vi "light_clock_data.vi"(11 "Pixel Colors":u32[](array[colorbox])) -> ()   [LabVIEW 2011]
uses:
  <vilib>/Rock Robotics/WPI/SPI/WPI_SPIDevRef.ctl
  <vilib>/vision/NI_Vision_Development_Module.lvlib
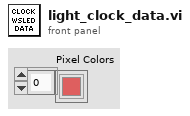
[diagram p1: front panel]
types:
  T1 = typedef "WPI_SPIDevRef.ctl" = cluster{"DevStatus":errorcluster}
  T2 = cluster{"Red (or Hue) value":u8, "Green (or Sat) value":u8, "Blue (or Light or Val) value":u8}
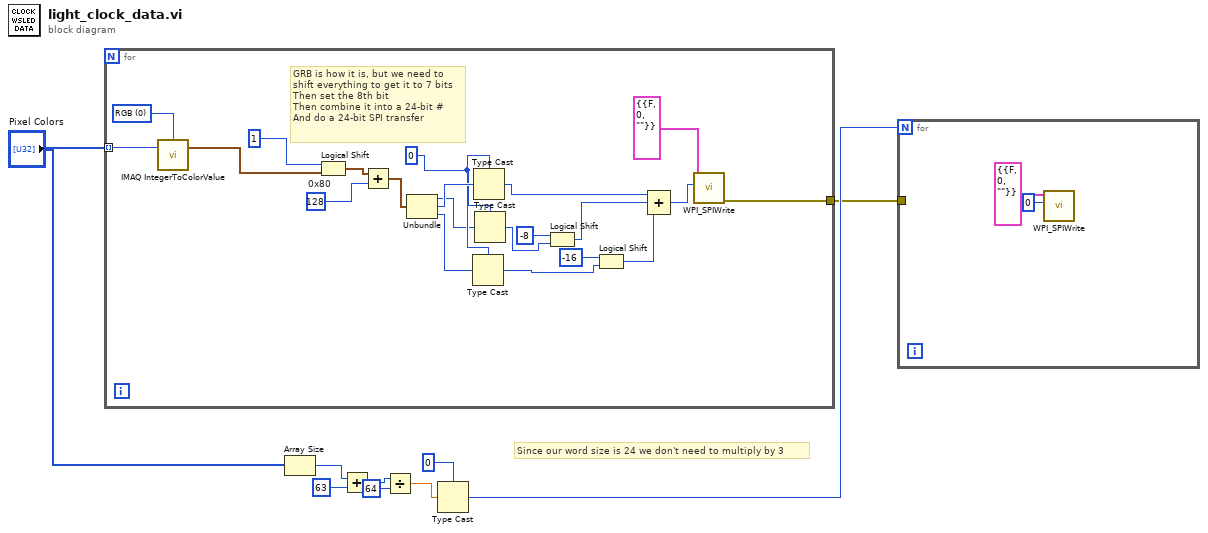
[diagram p0: block diagram]
diagram:
  # "Since our word size is 24 we don't need to multiply by 3"
  n1 = for {
    tunnel: "Pixel Colors" -> [w30] mode=indexing
    tunnel: [w10] -> w1
    w16 = u32 0
    w25 = u8 128  # 0x80
    w29 = u16 0 items=["RGB", "HSL", "HSV", "HSI"] ("Color Mode")
    # "GRB is how it is, but we need to\nshift everything to get it to 7 bits\nThen set the 8th bit\nThen combine it into a 24-bit #\nAnd do a 24-bit SPI transfer"
    n2 = call "IMAQ IntegerToColorValue"("U32 value"=w30, "Color Mode"=w29) -> ("Color Value"=w27:T2)  [unwired: 3 in, 3 out]
    n3 = Logical Shift(y=1, x=w27) -> (x << y=w26:T2)
    n4 = Add(x=w26, y=w25) -> (x+y=w19:T2)
    n5 = Unbundle(w19) -> ("Red (or Hue) value"=w15:u8, "Green (or Sat) value"=w18:u8, "Blue (or Light or Val) value"=w14:u8)
    n6 = Type Cast(type=w16, x=w14) -> (*(type *) &x=w12:u32)
    n7 = Type Cast(type=w16, x=w18) -> (*(type *) &x=w17:u32)
    n8 = Type Cast(type=w16, x=w15) -> (*(type *) &x=w13:u32)
    n9 = Logical Shift(y=i8 -8, x=w13) -> (x << y=w23:u32)
    n10 = Logical Shift(y=i8 -16, x=w12) -> (x << y=w22:u32)
    n11 = Compound Arithmetic op=ADD(w17, w23, w22) -> (w20:u32)
    n12 = call <vilib>:"WPI_SPIWrite.vi"("Data To Send"=w20, "SPIDevRef"=T1 {"DevStatus"={"status"=FALSE, "code"=0, "source"=""}}) -> ("error out"=w10:errorcluster)  [unwired: 8 in, 1 out]
  }
  n13 = Array Size(array="Pixel Colors") -> (size(s)=w8:i32)
  n14 = Add(x=w8, y=63) -> (x+y=w6:i32)
  n15 = Divide(x=w6, y=64) -> (x/y=w4:dbl)
  n16 = Type Cast(type=0 ("y"), x=w4) -> (*(type *) &x=w2:i32)
  n17 = for {
    N: w2 -> [_]
    tunnel: w1 -> [_]
    n18 = call <vilib>:"WPI_SPIWrite.vi"("Data To Send"=u32 0, "SPIDevRef"=T1 {"DevStatus"={"status"=FALSE, "code"=0, "source"=""}}) -> ()  [unwired: 8 in, 2 out]
  }
